vi "categorize_command.vi"(11 "command":string) -> (2 "HW":T1=enum."Unknown", 3 "command (out)":string)   [LabVIEW 2017]
uses:
  controls/HW_selection.ctl
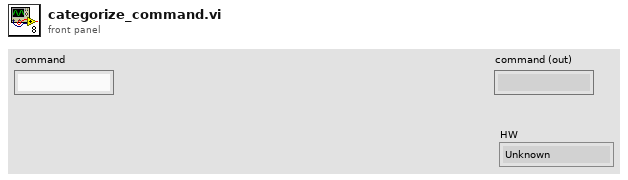
[diagram p1: front panel]
types:
  T1 = typedef "HW_selection.ctl" = enum16{"Sample Handler", "SQUID", "Degausser", "ARM", "IRM", "Robot", "System", "Unknown"}
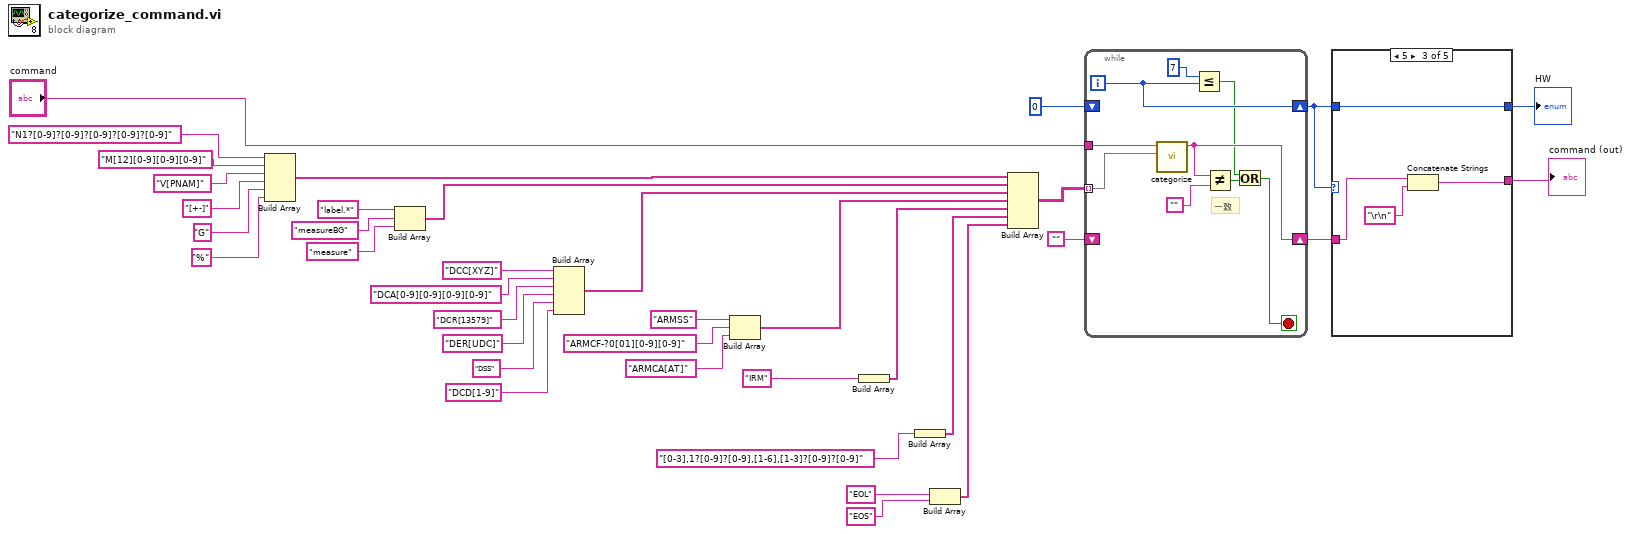
[diagram p0: block diagram]
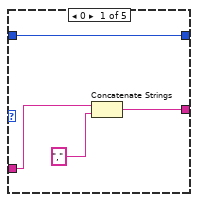
[diagram p2: hidden frame]
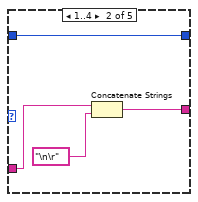
[diagram p3: hidden frame]
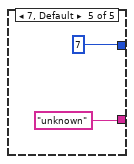
[diagram p5: hidden frame]
diagram:
  n1 = Build Array("N1?[0-9]?[0-9]?[0-9]?[0-9]?[0-9]", "M[12][0-9][0-9][0-9]", "V[PNAM]", "[+-]", "G", "%") -> (w24:string[])
  n2 = Build Array("label.*", "measureBG", "measure") -> (w23:string[])
  n3 = Build Array("DCC[XYZ]", "DCA[0-9][0-9][0-9][0-9]", "DCR[13579]", "DER[UDC]", "DSS", "DCD[1-9]") -> (w22:string[])
  n4 = Build Array("ARMSS", "ARMCF-?0[01][0-9][0-9]", "ARMCA[AT]") -> (w21:string[])
  n5 = Build Array("IRM") -> (w12:string[])
  n6 = Build Array("[0-3],1?[0-9]?[0-9],[1-6],[1-3]?[0-9]?[0-9]") -> (w14:string[])
  n7 = Build Array("EOL", "EOS") -> (w6:string[])
  n8 = Build Array(w24, w23, w22, w21, w12, w14, w6) -> (w20:string[][])
  n9 = while {
    tunnel: w20 -> [w45] mode=indexing
    tunnel: "command" -> [w46]
    shift-right: [w43] -> w11
    shift-left: "" -> [_]
    shift-right: [w41] -> w9
    shift-left: 0 -> [_]
    i -> [w41]
    stop <- w38 stop-if-true
    # "一致"
    n10 = call "categorize.vi"("候補配列（正規表現）"=w45, "入力文字列"=w46) -> ("結果"=w43:string)  [unwired: 9 in]
    n11 = Less Or Equal?(x=7, y=w41) -> (x <= y?=w39:bool)
    n12 = Not Equal?(x=w43, y="") -> (x != y?=w40:bool)
    n13 = Or(x=w39, y=w40) -> (x .or. y?=w38:bool)
  }
  n14 = case shown="5" w9 {
    tunnel: w11 -> [w50 w54 w57 w59 _]
    tunnel: [w48 w52 w55 w59 "unknown"] -> w10
    tunnel: w9 -> [w47 w51 w58 w60 _]
    tunnel: [w47 w51 w58 w60 7] -> w8
    frame 0 {
      n15 = Concatenate Strings(w50, ",") -> (w48:string)
    }
    frame 1..4 {
      n16 = Concatenate Strings(w54, "\n\r") -> (w52:string)
    }
    frame 5 {
      n17 = Concatenate Strings(w57, "\r\n") -> (w55:string)
    }
    frame 6 {
    }
    frame 7, Default {
    }
  }
  "HW" <- w8
  "command (out)" <- w10
